vi "Server.vi"() -> ()   [LabVIEW 2015]
panel:
  in  "Stop Sending":bool
  in  "Message":string
  out "Error out":errorcluster
  in  "Timeout [ms]\n (wait forever: -1)":i32=-1
  in  "Port":u16
  # "Server"
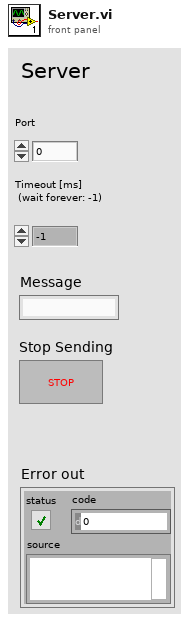
[diagram p1: front panel]
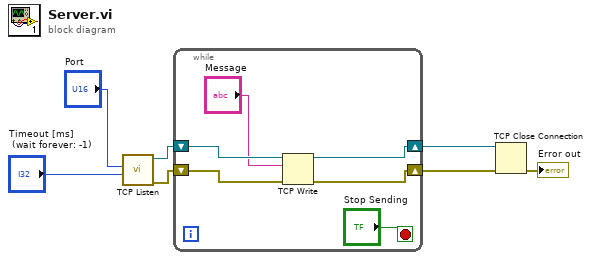
[diagram p0: block diagram]
diagram:
  n1 = call <vilib>:"TCP Listen.vi"("timeout ms (wait forever: -1)"="Timeout [ms]\n (wait forever: -1)", "port"="Port") -> ("error out"=w3:errorcluster, "connection ID"=w5:refnum<k5>)  [unwired: 5 in, 3 out]
  n2 = while {
    shift-right: [w12] -> w4
    shift-left: w5 -> [w13]
    shift-right: [w10] -> w2
    shift-left: w3 -> [w11]
    stop <- "Stop Sending" stop-if-true
    n3 = TCP Write(connection ID=w13, data in="Message", error in (no error)=w11) -> (connection ID out=w12:refnum<k5>, error out=w10:errorcluster)  [unwired: 1 in, 1 out]
  }
  n4 = TCP Close Connection(connection ID=w4, error in (no error)=w2) -> (error out=→"Error out":errorcluster)  [unwired: 1 in, 1 out]
